vi "to string 3.0.vi"(8 "error in":errorcluster, 10 "data in":string, 11 "Shared Memory configuration in":refnum<class "Shared Memory configuration.lvclass">) -> (0 "error out":errorcluster, 2 "data out":string, 3 "Shared Memory configuration out":refnum<class "Shared Memory configuration.lvclass">)   [LabVIEW 2014, in "Shared Memory configuration.lvclass"]
uses:
  Shared Memory configuration.lvclass
  Shared Memory configuration.lvclass/Shared Memory configuration.ctl
  <vilib>/NI/Configuration Framework/serializable configuration/NISE_CEF_serializable configuration.lvclass
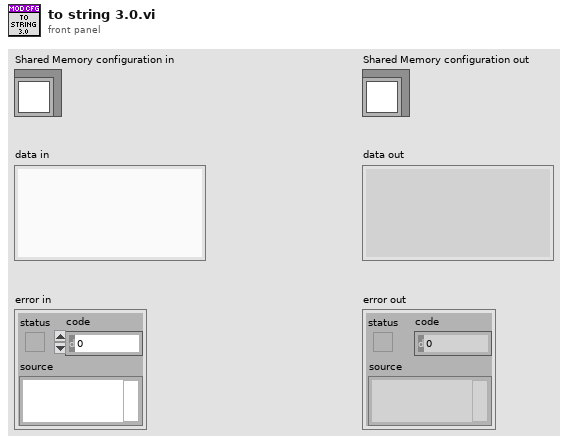
[diagram p1: front panel]
types:
  T1 = typedef "Shared Memory configuration.lvclass/sync item.ctl" = cluster{"mechanism":T2, "name":string}
  T2 = typedef "Shared Memory configuration.lvclass/sync mechanism.ctl" = enum16{"Semaphore"}
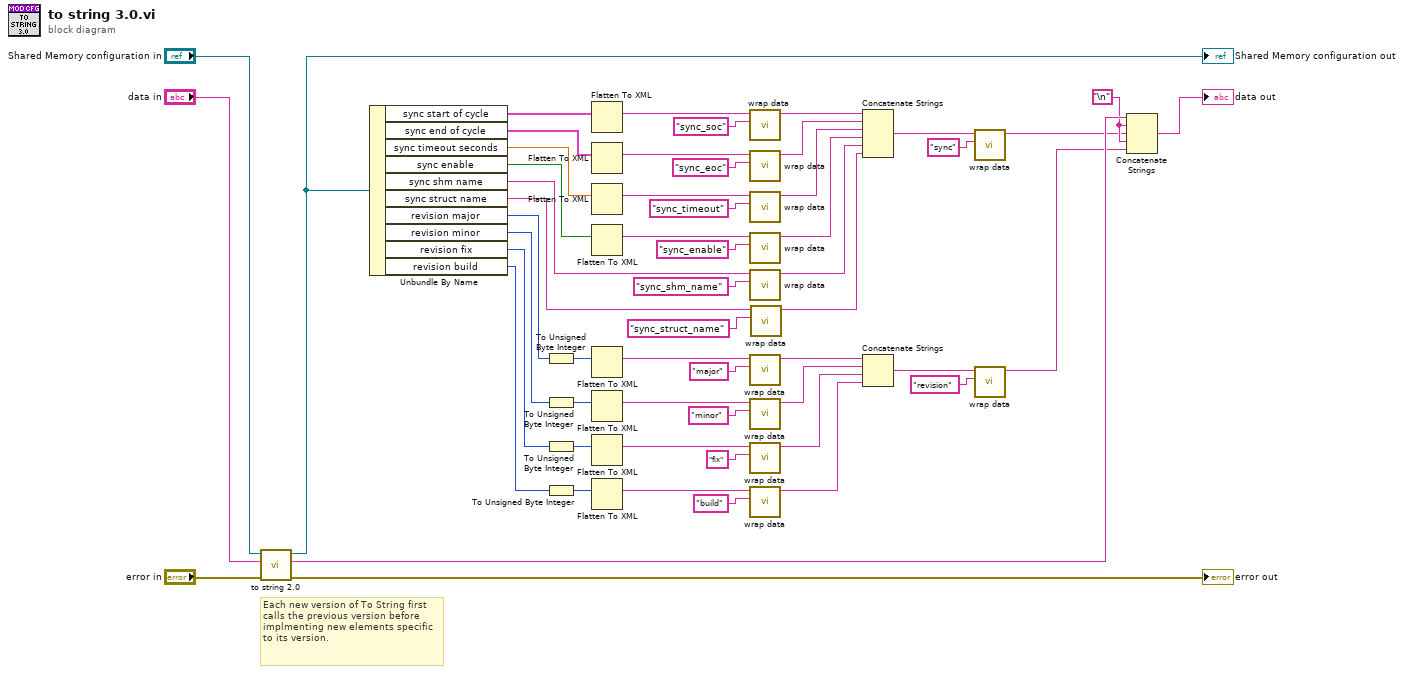
[diagram p0: block diagram]
diagram:
  w9 = "\n"
  # "Each new version of To String first calls the previous version before implmenting new elements specific to its version."
  n1 = call "to string 2.0.vi"("error in"="error in", "data in"="data in", "Shared Memory configuration in"="Shared Memory configuration in") -> ("error out"=→"error out":errorcluster, "data out"=w13:string, "Shared Memory configuration out"=w10:refnum<class "Shared Memory configuration.lvclass">)  [unwired: 6 in]
  "Shared Memory configuration out" <- w10
  n2 = Unbundle By Name(w10) -> ("sync start of cycle"=w17:T1[], "sync end of cycle"=w54:T1[], "sync timeout seconds"=w49:dbl, "sync enable"=w46:bool, "sync shm name"=w43:string, "sync struct name"=w12:string, "revision major"=w21:u16, "revision minor"=w34:u16, "revision fix"=w2:u16, "revision build"=w1:u16)
  n3 = To Unsigned Byte Integer(number=w21) -> (unsigned 8bit integer=w6:u8)
  n4 = To Unsigned Byte Integer(number=w34) -> (unsigned 8bit integer=w5:u8)
  n5 = To Unsigned Byte Integer(number=w2) -> (unsigned 8bit integer=w3:u8)
  n6 = To Unsigned Byte Integer(number=w1) -> (unsigned 8bit integer=w4:u8)
  n7 = Flatten To XML(anything=w17) -> (xml string=w53:string)
  n8 = Flatten To XML(anything=w54) -> (xml string=w51:string)
  n9 = Flatten To XML(anything=w49) -> (xml string=w48:string)
  n10 = Flatten To XML(anything=w46) -> (xml string=w45:string)
  n11 = Flatten To XML(anything=w6) -> (xml string=w38:string)
  n12 = Flatten To XML(anything=w5) -> (xml string=w35:string)
  n13 = Flatten To XML(anything=w3) -> (xml string=w36:string)
  n14 = Flatten To XML(anything=w4) -> (xml string=w37:string)
  n15 = call <vilib>:"wrap data.vi"("identifier"="sync_soc", "data to wrap"=w53) -> ("wrapped data"=w32:string)  [unwired: 9 in]
  n16 = call <vilib>:"wrap data.vi"("identifier"="sync_eoc", "data to wrap"=w51) -> ("wrapped data"=w31:string)  [unwired: 9 in]
  n17 = call <vilib>:"wrap data.vi"("identifier"="sync_timeout", "data to wrap"=w48) -> ("wrapped data"=w30:string)  [unwired: 9 in]
  n18 = call <vilib>:"wrap data.vi"("identifier"="sync_enable", "data to wrap"=w45) -> ("wrapped data"=w29:string)  [unwired: 9 in]
  n19 = call <vilib>:"wrap data.vi"("identifier"="sync_shm_name", "data to wrap"=w43) -> ("wrapped data"=w28:string)  [unwired: 9 in]
  n20 = call <vilib>:"wrap data.vi"("identifier"="major", "data to wrap"=w38) -> ("wrapped data"=w26:string)  [unwired: 9 in]
  n21 = call <vilib>:"wrap data.vi"("identifier"="minor", "data to wrap"=w35) -> ("wrapped data"=w25:string)  [unwired: 9 in]
  n22 = call <vilib>:"wrap data.vi"("identifier"="fix", "data to wrap"=w36) -> ("wrapped data"=w24:string)  [unwired: 9 in]
  n23 = call <vilib>:"wrap data.vi"("identifier"="build", "data to wrap"=w37) -> ("wrapped data"=w23:string)  [unwired: 9 in]
  n24 = call <vilib>:"wrap data.vi"("identifier"="sync_struct_name", "data to wrap"=w12) -> ("wrapped data"=w18:string)  [unwired: 9 in]
  n25 = Concatenate Strings(w32, w31, w30, w29, w28, w18) -> (w27:string)
  n26 = Concatenate Strings(w26, w25, w24, w23) -> (w22:string)
  n27 = call <vilib>:"wrap data.vi"("identifier"="sync", "data to wrap"=w27) -> ("wrapped data"=w8:string)  [unwired: 9 in]
  n28 = call <vilib>:"wrap data.vi"("identifier"="revision", "data to wrap"=w22) -> ("wrapped data"=w7:string)  [unwired: 9 in]
  n29 = Concatenate Strings(w13, w9, w8, w9, w7) -> (→"data out":string)
